vi "Main Controler.vi"() -> ()   [LabVIEW 2022 SP3]
uses:
  Controls/Display Loop ctl.ctl
  Loop.ctl
  Controls/ALL Health.ctl
  cd6b9e46-59f8-41b3-9490-225fb67d1ba0.vi
  1b3de88b-dec3-4abe-965c-7ad6896efe13.vi
  9936e6a7-bc3d-4afe-8410-a89b98546ed9.vi
  d1ab7018-2df1-4ffb-970b-af0fe01cb293.vi
  e0eb6b05-03bb-4813-a05d-282ab3cd3a22.vi
  ecf1675c-338f-4a89-ac69-4cdab471b100.vi
  ca0a8722-a5c4-4655-b82c-d313b5c34e14.vi
  c976ff62-2192-4a2c-b2cc-abbf70db85cd.vi
  943ba9a9-8a3c-4e90-9b72-098ad84989a2.vi
  675b6325-e57b-42b8-b386-55e59851567e.vi
  d7703bda-d248-4b1e-9ee4-ce44b9949d59.vi
  ad1d9b89-0aa4-4254-89c1-c2ee87c320aa.vi
  35d283f9-0e0c-41d3-ba70-7538f373975d.vi
  c92325a5-4571-45f9-94fe-0f0a9663467d.vi
  6D_Global.vi
  8e23ed98-7719-4f36-858a-146910f058b4.vi
panel:
  out "OUT_D_PT":dbl format="%.2g"
  out "AI 1kHZ HS":bool
  out "D_PT_2":dbl format="%.2f"
  out "D_RTD_1":dbl format="%#.2g"
  out "D_PT_1":dbl format="%.2g"
  out "M_RTD_1":dbl format="%#.2g"
  out "M_PT_1":dbl format="%.2g"
  out "OUT_D_RTD":dbl format="%#.2g"
  out "IN_D_RTD":dbl format="%#.2g"
  out "D_RTD_2":dbl format="%#.2g"
  out "IN_D_PT":dbl format="%.2g"
  out "AI 20kHZ HS":bool
  out "Vdc":dbl
  out "Ic_Unbal":bool
  out "Ib_Unbal":bool
  out "Ia_Unbal":bool
  out "Overall Unbal":bool
  out "Ic_G":bool
  out "Ib_G":bool
  out "Ia_G":bool
  out "IDC":bool
  out "Ic":bool
  out "Ib":bool
  out "Ia":bool
  in  "Unbal Threshold":dbl
  in  "10 SAMPLES _G":dbl
  in  "2 SAMPLES_G":dbl
  in  "Log Period":dbl=900.0
  out "DO HS":bool
  out "Idc_G":dbl
  out "Vdc_G":dbl
  out "Hc_G":bool=TRUE
  out "Hb_G":bool=TRUE
  out "Ha_G":bool=TRUE
  out "Ic_G":dbl
  out "Ib_G":dbl
  out "Ia_G":dbl
  out "Vca_G":dbl
  out "Vbc_G":dbl
  out "Vab_G":dbl
  in  "Update RTD Offset_G 2":bool
  in  "V-Ref_B":dbl=3.306
  in  "RTD 6 Offset_B":dbl=1.432
  in  "RTD 5 Offset_B":dbl=1.432
  in  "RTD 4 Offset_B":dbl=1.427
  in  "RTD 3 Offset_B":dbl=1.421
  in  "RTD 2 Offset_B":dbl=1.429
  in  "RTD 1 Offset_B":dbl=1.429
  out "RTD  6":dbl format="%#_f "
  out "RTD  5":dbl format="%#_f "
  out "RTD  4":dbl format="%#_f "
  out "RTD  3":dbl format="%#_f "
  out "RTD  2":dbl format="%#_f "
  out "RTD  1":dbl format="%#_f "
  out "AI HS":bool
  in  "Update RTD Offset_G":bool
  in  "V-Ref_G":dbl=3.306
  in  "RTD 6 Offset_G":dbl=1.432
  in  "RTD 5 Offset_G":dbl=1.432
  in  "RTD 4 Offset_G":dbl=1.427
  in  "RTD 3 Offset_G":dbl=1.421
  in  "RTD 2 Offset_G":dbl=1.429
  in  "RTD 1 Offset_G":dbl=1.429
  out "LOG HS":bool
  in  "Datalog Prefix":string
  in  "Activate Task 2":T1
  in  "Update RTD Offset":bool
  in  "V-Ref":dbl=3.29
  in  "RTD 6 Offset":dbl
  in  "RTD 5 Offset":dbl
  in  "RTD 4 Offset":dbl
  in  "RTD 3 Offset":dbl
  in  "RTD 2 Offset":dbl
  in  "RTD 1 Offset":dbl
  out "DAQ Idc":dbl
  out "M-STATE FB":bool
  out "RUN DUTY RATIO":dbl format="%#_6f"
  out "IDC":dbl format="%#_f "
  out "Idc M-Avg":dbl format="%#_f "
  out "VOLTAGE SPEED":dbl format="%#_f "
  out "HALL SPEED":dbl format="%#_f "
  out "SECTOR":dbl format="%#_f "
  out "VDC":dbl format="%#_f "
  out "DIRECTION":string
  out "RUN ACK":bool
  out "Hc":bool=TRUE
  out "Hb":bool=TRUE
  out "Ha":bool=TRUE
  out "Ic":dbl
  out "Ib":dbl
  out "Ia":dbl
  out "Vca":dbl
  out "Vbc":dbl
  out "Vab":dbl
  out "Power Failure":bool
  out "M-S Failure":bool=TRUE
  out "PPSU Alarm":bool
  out "Over Voltage":bool
  out "Over Current":bool
  out "Over Power":bool
  in  "IDC":dbl
  in  "10 SAMPLES":dbl
  in  "2 SAMPLES":dbl
  out "RUN DUTY RATIO":dbl format="%#_6f"
  out "M-STATE FB":bool
  out "IDC":dbl format="%#_f "
  out "Idc M-Avg":dbl format="%#_f "
  out "VOLTAGE SPEED":dbl format="%#_f "
  out "HALL SPEED":dbl format="%#_f "
  out "SECTOR":dbl format="%#_f "
  out "VDC":dbl format="%#_f "
  out "DIRECTION":string
  out "RUN ACK":bool
  in  "PPSU IP":u8[](array[numeric])=[192, 168, 1, 120]
  in  "Enable PPSU":bool
  out "PPSU HS":bool
  in  "MS initialise":bool
  in  "PPSU ACK Alarm":bool
  out "PPSU 2 HS":bool
  out "VOLTAGE":string
  out "CURRENT":string
  out "POWER":string
  in  "DC OFF 2":bool
  in  "DC ON 2":bool
  in  "Motor Off":bool
  in  "DC OFF":bool
  in  "Motor On":bool
  in  "DC ON":bool
  out "E3-L-RTD":bool
  out "E3-A-RTD":bool
  out "E2-L-RTD":bool
  out "E5 - RTD":bool
  out "E2-RTD":bool
  out "E1-RTD":bool
  out "E1-MFB":bool
  out "E2-MFB":bool
  out "E2-A-MFB":bool
  out "E2-L-MFB":bool
  out "E3-A-MFB":bool
  out "E3-L-MFB":bool
  in  "Disconnect Drive":bool
  in  "Connect Drive":bool
  in  "Port Config File":path=path "C:/Users/Karishmaa- LabVIEW/Desktop/V1.0 Drive6_Control_Monitor/Data/Port ID Config .csv"
  in  "GD ON":bool
  in  "GD OFF":bool
  out "RTD  6":dbl format="%#_f "
  out "RTD  5":dbl format="%#_f "
  out "RTD  4":dbl format="%#_f "
  out "RTD  3":dbl format="%#_f "
  out "RTD  2":dbl format="%#_f "
  out "RTD  1":dbl format="%#_f "
  out "RTD 6":dbl format="%#_f "
  out "RTD  5":dbl format="%#_f "
  out "RTD  4":dbl format="%#_f "
  out "RTD 3":dbl format="%#_f "
  out "RTD  2":dbl format="%#_f "
  out "RTD  1":dbl format="%#_f "
  in  "Update PPSU settings":bool
  in  "PPSU-SETTINGS":T2 {"SET POWER" format="%#_g W"; "SET CURRENT" format="%#_g A"; "SET VOLT" format="%#_g V"; "OPP" format="%#_g W"; "OCP" format="%#_g A"; "OVP" format="%#_g V"}
  in  "Update E1A":bool
  in  "MOTOR":T3 {"M-STATE" format="%#_g "; "DC LIMIT" format="%#_g A"; "RAMP DOWN" format="%#_g Sec"; "RAMP UP" format="%#_g Sec"; "SWITCHING FREQ" format="%#_g Hz"}
  in  "DO CONFIG":cluster{"NAME":string, "CHANNEL NAME":tag}[](array[cluster])
  out "RTD  30":dbl format="%#_f "
  out "RTD  29":dbl format="%#_f "
  out "RTD  28":dbl format="%#_f "
  out "RTD  27":dbl format="%#_f "
  out "RTD  26":dbl format="%#_f "
  out "RTD  25":dbl format="%#_f "
  out "RTD  24":dbl format="%#_f "
  out "RTD  23":dbl format="%#_f "
  out "RTD  22":dbl format="%#_f "
  out "RTD  21":dbl format="%#_f "
  out "RTD  20":dbl format="%#_f "
  out "RTD  19":dbl format="%#_f "
  out "RTD  18":dbl format="%#_f "
  out "RTD  17":dbl format="%#_f "
  out "RTD  16":dbl format="%#_f "
  out "RTD  15":dbl format="%#_f "
  out "RTD  14":dbl format="%#_f "
  out "RTD  13":dbl format="%#_f "
  out "RTD  12":dbl format="%#_f "
  out "RTD  11":dbl format="%#_f "
  out "RTD  10":dbl format="%#_f "
  out "RTD  9":dbl format="%#_f "
  out "RTD  8":dbl format="%#_f "
  out "RTD  7":dbl format="%#_f "
  out "FREQUENCY  2":dbl format="%#_f "
  out "VDC  3":dbl format="%#_f "
  out "IDC  3":dbl format="%#_f "
  out "MOV-IDC  2":dbl format="%#_f "
  out "M-STATE  2":dbl format="%#_f "
  out "DIRECTION  2":string
  out "SPEED 5":dbl format="%#_f r/m"
  out "RUN ACK 5":bool
  out "FREQUENCY  2":dbl format="%#_f "
  out "VDC 2":dbl format="%#_f "
  out "IDC  3":dbl format="%#_f "
  out "MOV-IDC  2":dbl format="%#_f "
  out "M-STATE  2":dbl format="%#_f "
  out "DIRECTION  2":string
  out "SPEED 4":dbl format="%#_f r/m"
  out "RUN ACK 4":bool
  out "FREQUENCY  2":dbl format="%#_f "
  out "VDC  2":dbl format="%#_f "
  out "IDC 2":dbl format="%#_f "
  out "MOV-IDC  2":dbl format="%#_f "
  out "M-STATE  2":dbl format="%#_f "
  out "DIRECTION  2":string
  out "SPEED 3":dbl format="%#_f r/m"
  out "RUN ACK 3":bool
  out "FREQUENCY  2":dbl format="%#_f "
  out "VDC  2":dbl format="%#_f "
  out "IDC  2":dbl format="%#_f "
  out "MOV-IDC  2":dbl format="%#_f "
  out "M-STATE  2":dbl format="%#_f "
  out "DIRECTION  2":string
  out "SPEED 2":dbl format="%#_f r/m"
  out "RUN ACK 2":bool
  in  "Start DAQ":bool
  in  "Stop DAQ":bool
  in  "Start Log":bool
  in  "Stop Log":bool
  in  "Continuous Log?":bool
  in  "Activate Task":T4
  in  "Exit":bool
  # "DRIVE PARMETERS SETTINGS"
  # "*Select section to set parameters"
  # "DRIVE-3- CONTROL & MONITORING SCREEN"
  # "VERSION 1.0"
  # "ACTIVE PORTS"
  # "MOTOR FEEDBACK DATA"
  # "PPSU DATA"
  # "PPSU HS"
  # "DAQ & LOG SETTINGS"
  # "MOTOR"
  # "GENERATOR"
  # "PROPULSION"
  # "PPSU-2 HS"
  # "PROTECTION"
  # "MCU RESET"
  # "E2-ATF MOTOR FEEDBACK DATA"
  # "E2-LOX MOTOR FEEDBACK DATA"
  # "E3-ATF MOTOR FEEDBACK DATA"
  # "E3-ATF MOTOR FEEDBACK DATA"
  # "E2-ATF TEMPRATURE DATA"
  # "E2-LOX TEMPRATURE DATA"
  # "E3-ATF TEMPRATURE DATA"
  # "E3-LOX TEMPRATURE DATA"
  # "BEARING TEMPRATURE DATA"
  # "E1-LOX"
  # "E1-ATF"
  # "E2-ATF"
  # "E2-LOX"
  # "E3-ATF"
  # "E3-LOX"
  # "GENERATOR FEEDBACK DATA"
  # "GENERATOR TEMPRATURE DATA"
  # "MOTOR TEMPRATURE DATA"
  # "GNIKUL"
  # "Drive 1"
  # "Drive 2"
  # "Drive 3"
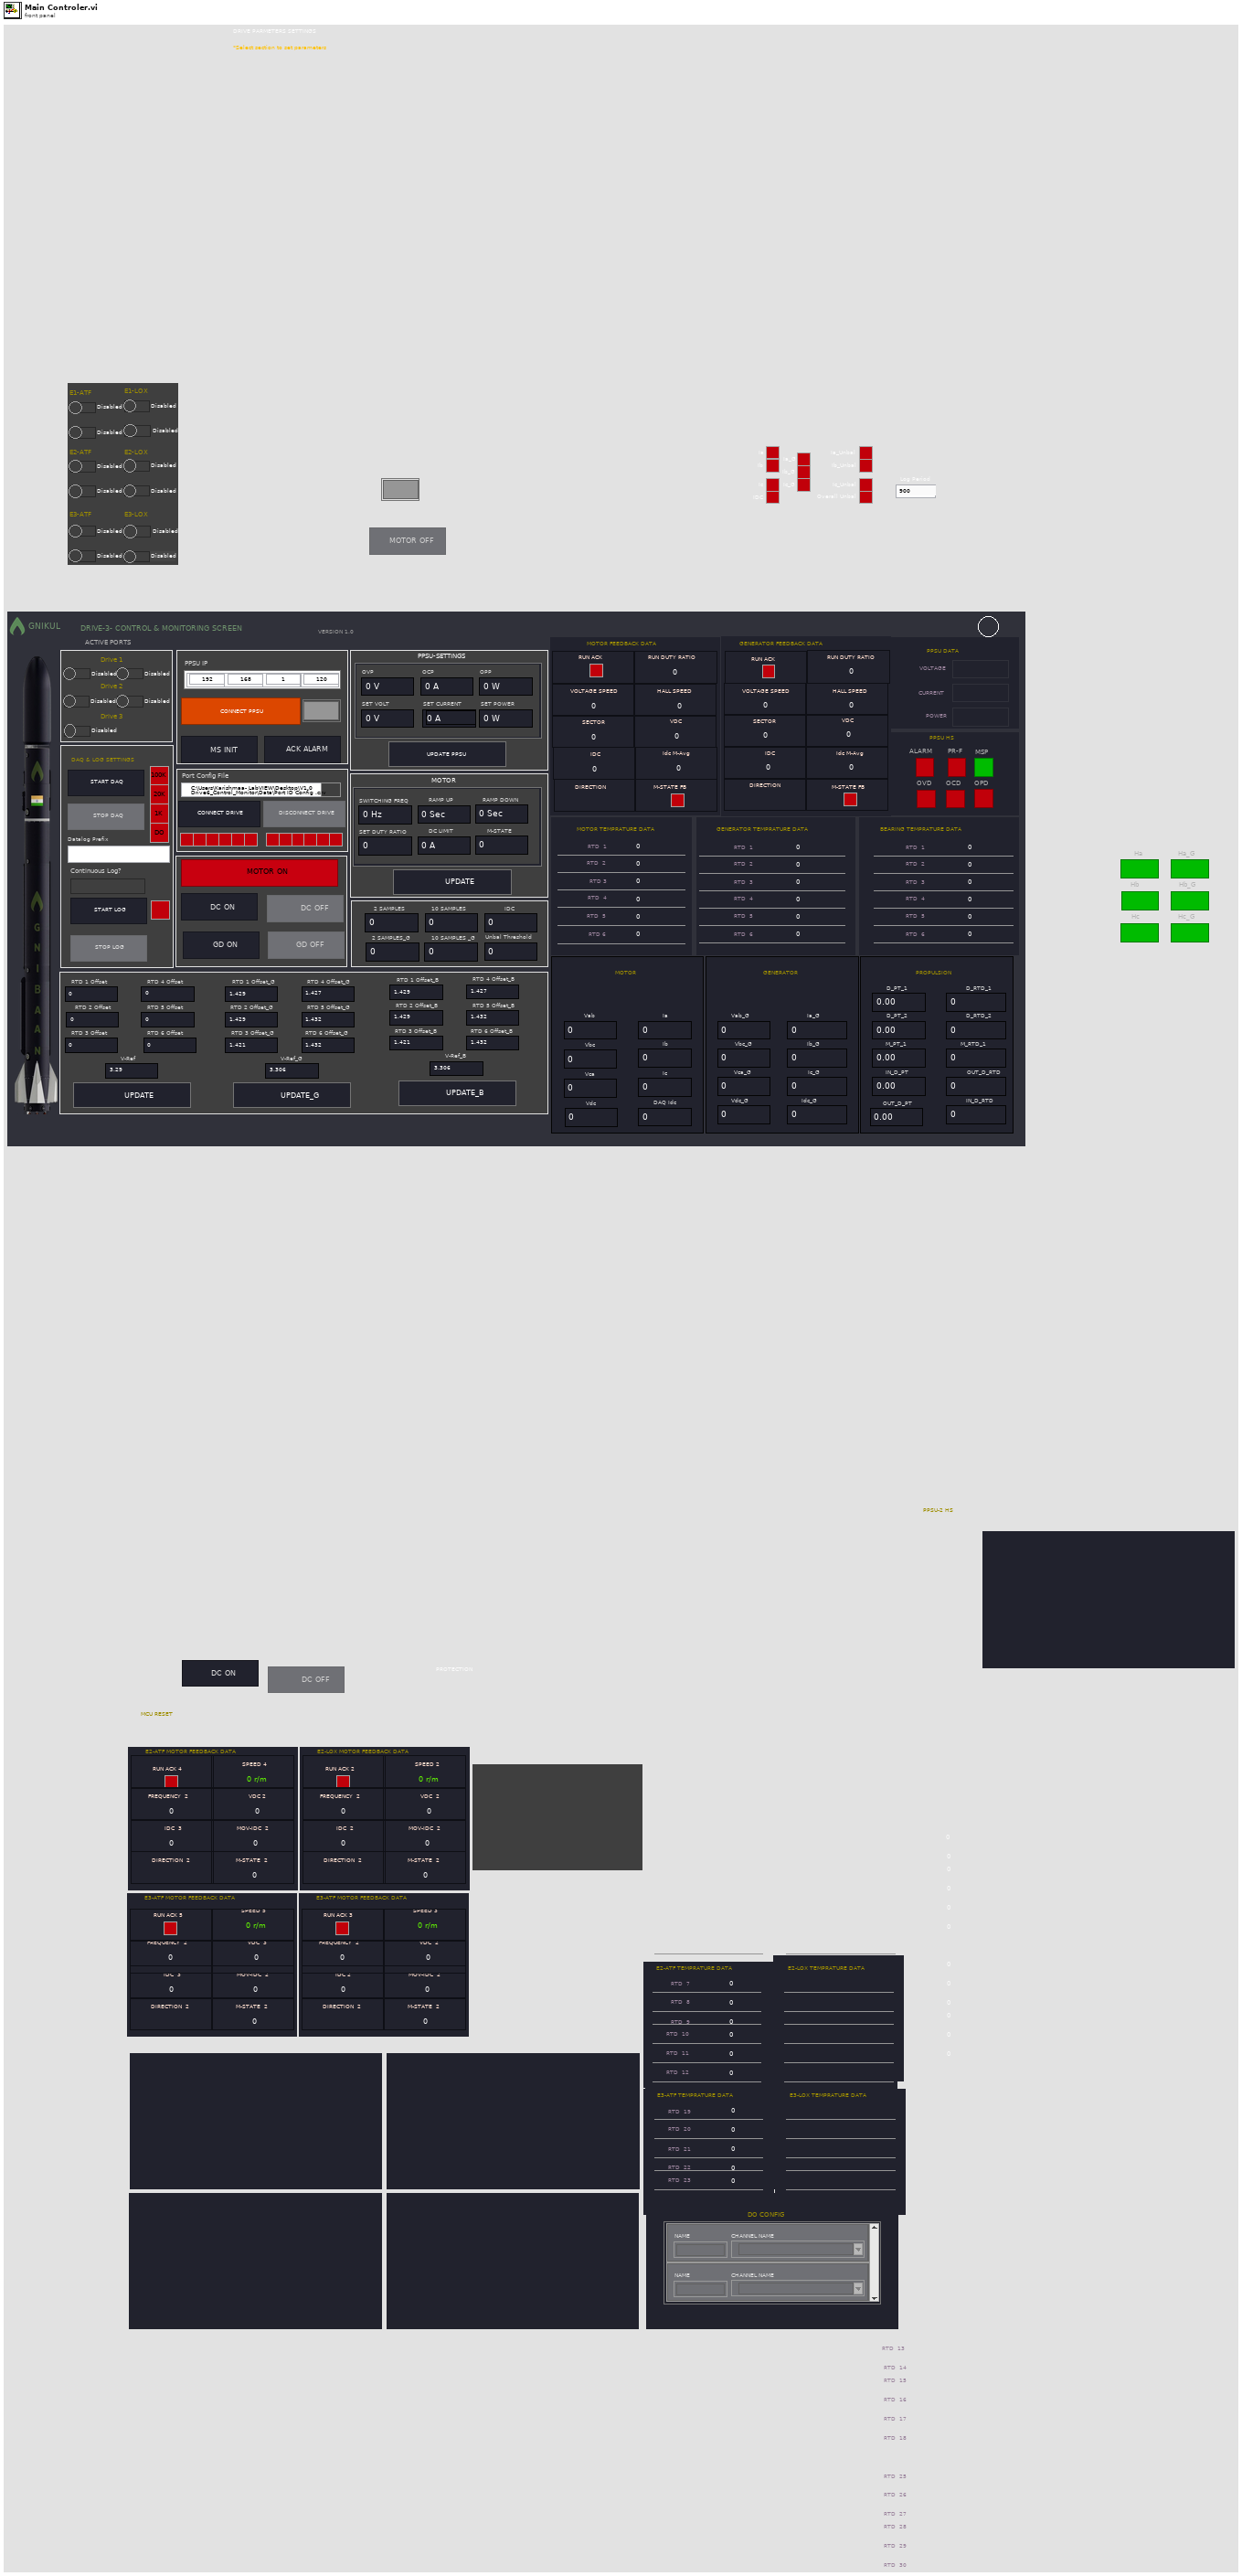
[diagram p1: front panel]
types:
  T1 = cluster{"ETH_1":bool, "ETH_2":bool, "ETH_3":bool, "ETH_4":bool, "ETH_5":bool, "ETH_6":bool, "ETH_7":bool, "ETH_8":bool, "ETH_9":bool, "ETH_10":bool, "ETH_11":bool, "ETH_12":bool}
  T2 = cluster{"OPP":dbl, "OVP ":dbl, "OCP":dbl, "SET VOLT":dbl, "SET CURRENT":dbl, "SET POWER":dbl}
  T3 = cluster{"SWITCHING FREQ":dbl, "RAMP UP":dbl, "RAMP DOWN":dbl, "SET DUTY RATIO":dbl, "DC LIMIT":dbl, "M-STATE":dbl}
  T4 = cluster{"ETH_1":bool, "ETH_2":bool, "ETH_3":bool, "ETH_4":bool, "ETH_3 2":bool}
  T5 = enum16{"Init", "Read 'All'", "Read 'n'", "Read '1'", "Write '1'", "Write 'n'", "Write 'All'"}
  T6 = typedef "Display Loop ctl.ctl" = enum16{"Motor", "RTD", "All Health", "PPSU"}
  T7 = enum16{"Init", "EnQ '1'", "EnQ 'n'", "EnQ Opp", "DeQ", "Flush", "Close"}
  T8 = cluster{"Device information":string[], "Device information array":string[][], "PPSU IP String":string}
  T9 = cluster{"ETH_1":bool, "ETH_2":bool, "ETH_3":bool, "ETH_4":bool, "ETH_5":bool}
  T10 = enum8{"Enabled", "Disabled", "Disabled and Grayed Out"}[]
  T11 = typedef "All Queue Ref.ctl" = cluster{"MFB":cluster{"ETH_1 E1A_MFB":refnum<queue>, "ETH_3 E1L_MFB":refnum<queue>, "ETH_5 E2A_MFB":refnum<queue>, "ETH_7 E2L_MFB":refnum<queue>, "ETH_9 E3A_MFB":refnum<queue>, "ETH_11 E3L_MFB":refnum<queue>}, "RTD":cluster{"ETH_2 E1A_RTD ":refnum<queue>, "ETH_4 E1L_RTD ":refnum<queue>, "ETH_6 E2A_RTD ":refnum<queue>, "ETH_8 E2L_RTD ":refnum<queue>, "ETH_10 E3A_RTD ":refnum<queue>, "ETH_12 E3L_RTD ":refnum<queue>}, "DO DAQ":refnum<queue>, "PPSU 1 Data":refnum<queue>, "PPSU 2 Data":refnum<queue>, "AI DAQ RMS DATA":refnum<queue>, "AI DAQ RAW DATA":refnum<queue>, "DI DAQ":refnum<queue>, "AI Propulsion RAW DAQ Data":refnum<queue>, "AI Propulsion RMS DAQ Data":refnum<queue>, "AI Vibration DAQ Data":refnum<queue>}
  T12 = typedef "ALL Health.ctl" = enum16{"AI HS", "AI Vibration HS", "AI Propulsion HS", "DO HS", "Datalog HS", "PPSU HS", "ETH_1 DAQ", "ETH_1 RTD", "ETH_2 DAQ", "ETH_2 RTD", "ETH_5 RTD"}
  T13 = cluster{"Run ACK":bool, "RDR":dbl, "Sector":dbl, "Halls Speed":dbl, "Mode":bool, "Voltage Speed":dbl, "Direction":string, "IDC":dbl, "Movable average":dbl, "VDC":dbl}
  T14 = cluster{"Alarm":bool, "Power Fail":bool, "OVD":bool, "OCD":bool, "OPD":bool, "MSP":bool}
  T15 = typedef "Loop.ctl" = enum16{"ETH_1", "ETH_2", "ETH_3", "ETH_4", "ETH_5", "ETH_6", "ETH_7", "ETH_8", "ETH_9", "ETH_10", "ETH_11", "ETH_12"}
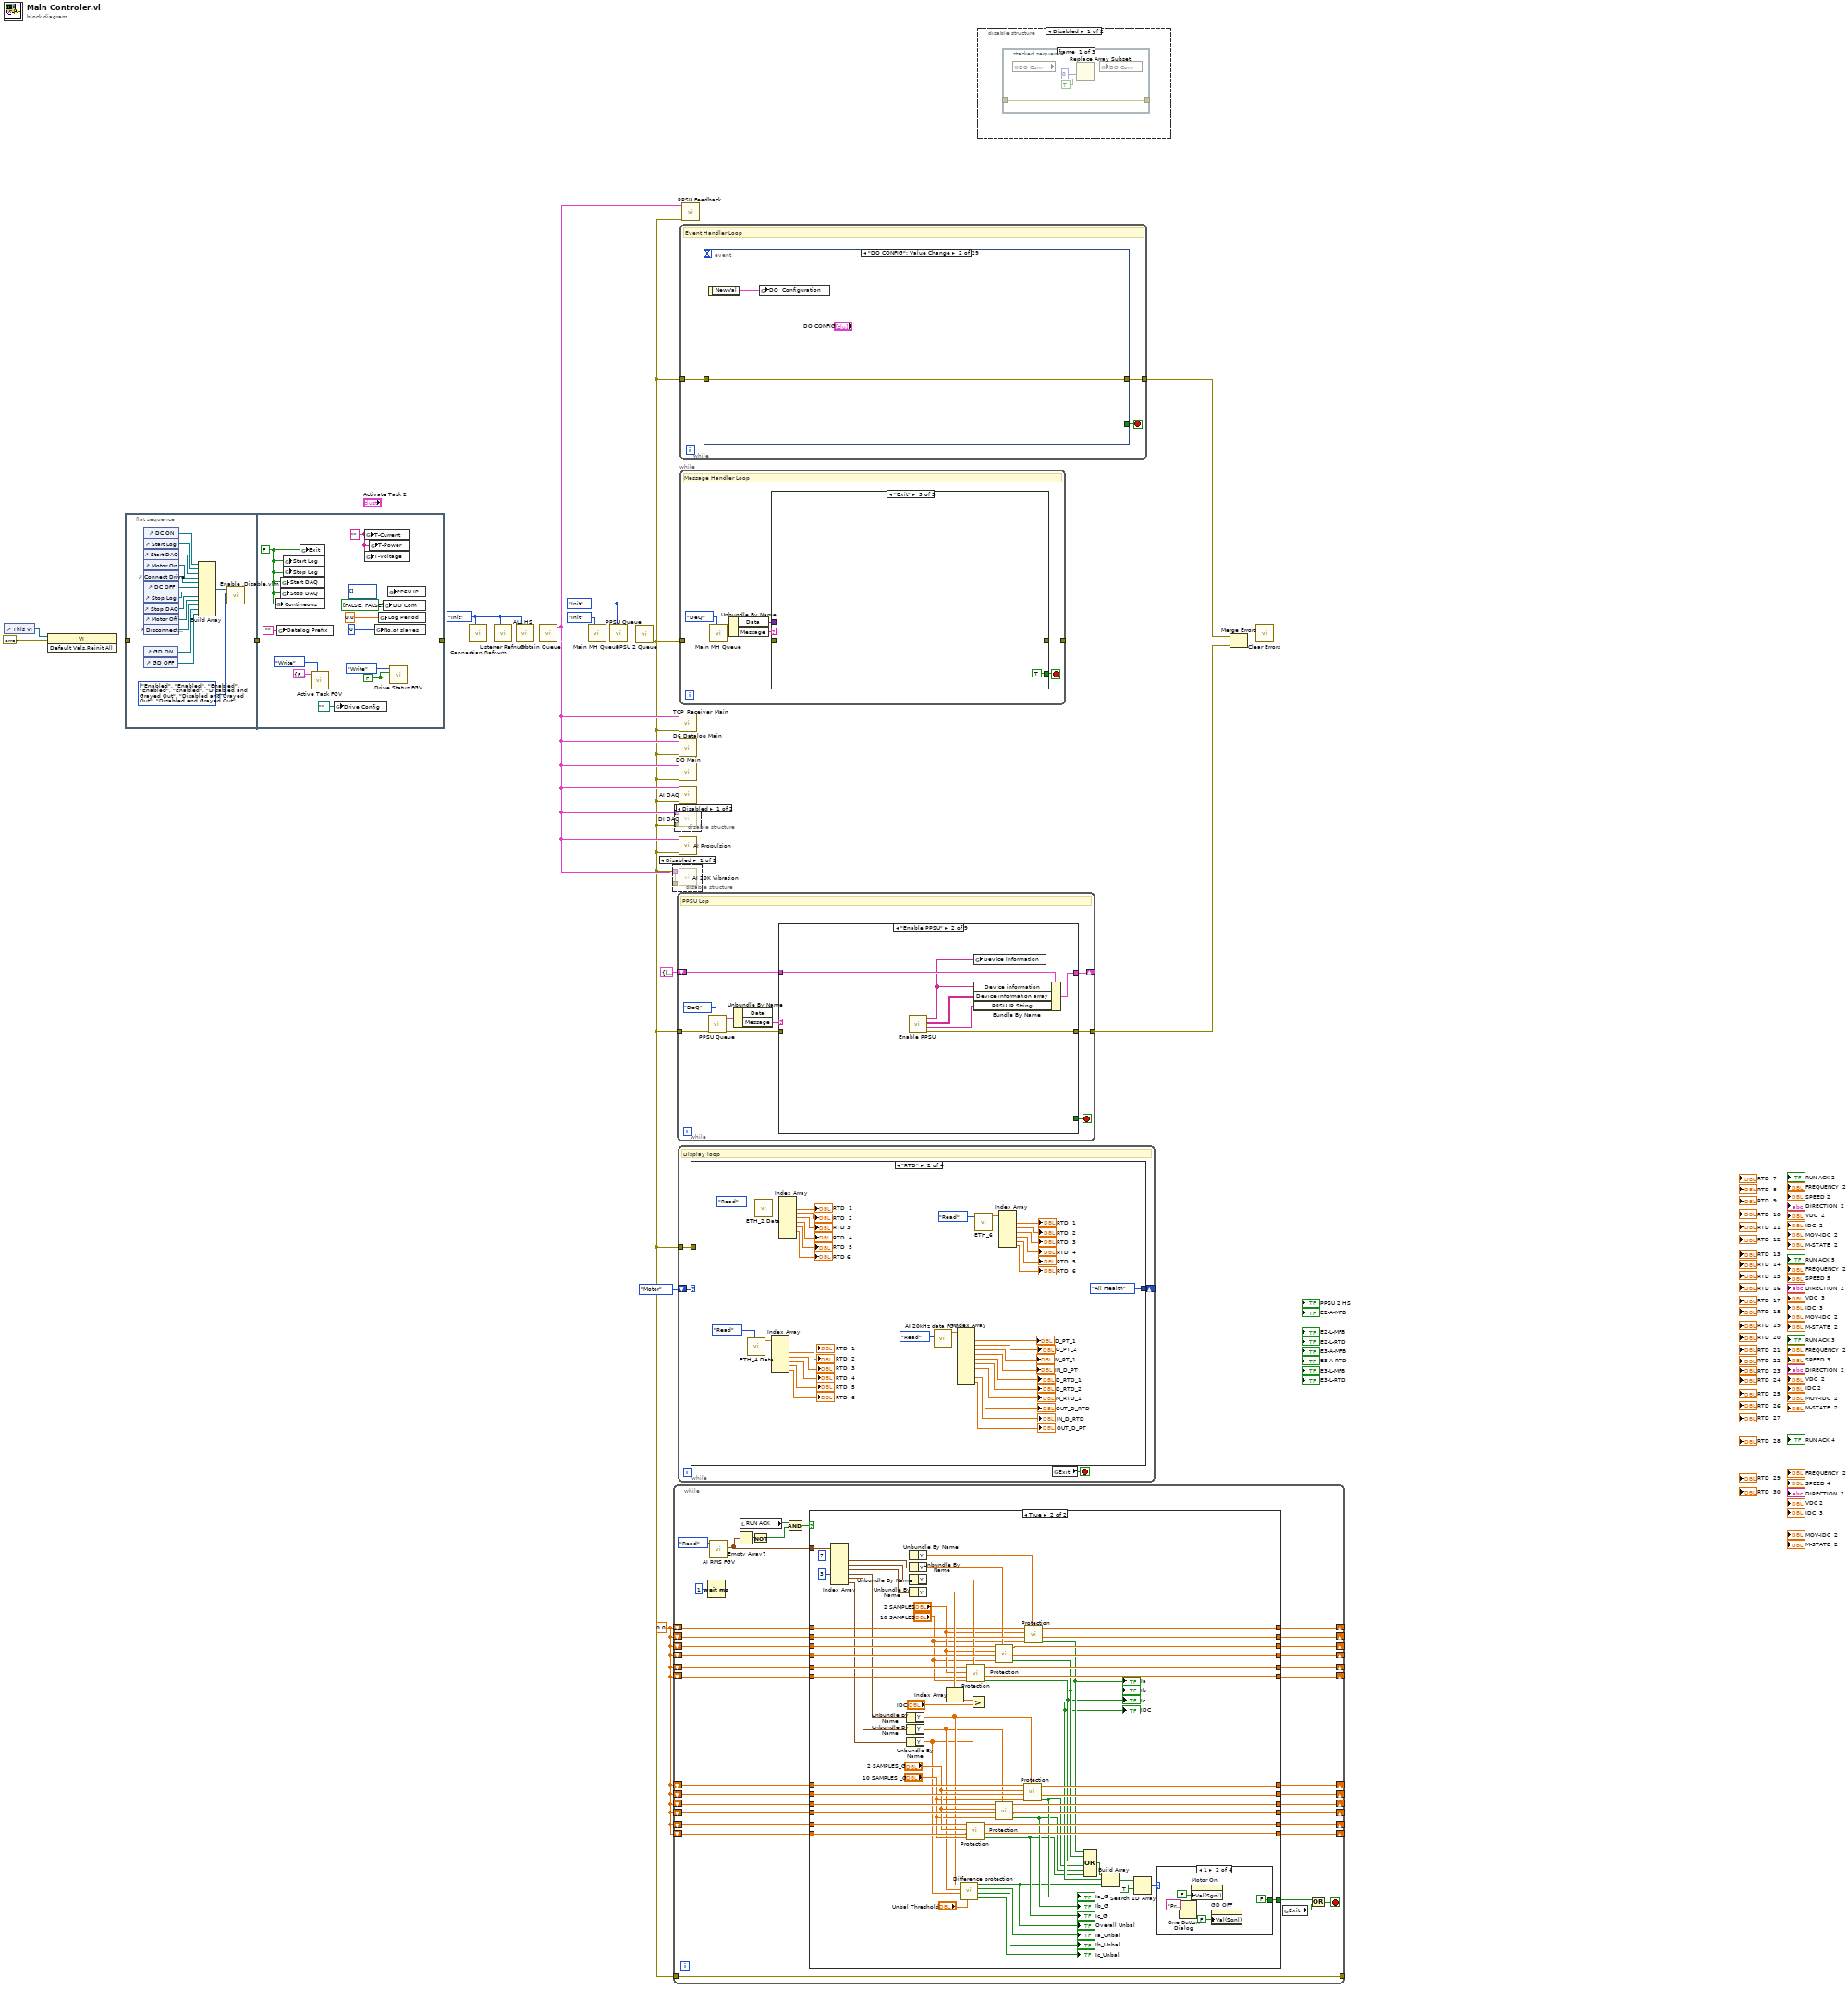
[diagram p0: block diagram]
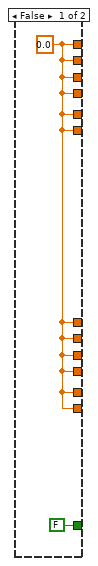
[diagram p4: hidden frame]
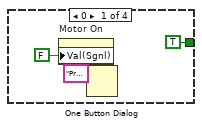
[diagram p5: hidden frame]
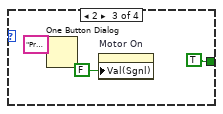
[diagram p6: hidden frame]
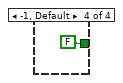
[diagram p7: hidden frame]
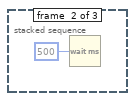
[diagram p8: hidden frame]
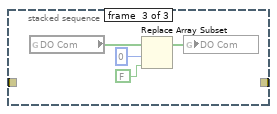
[diagram p9: hidden frame]
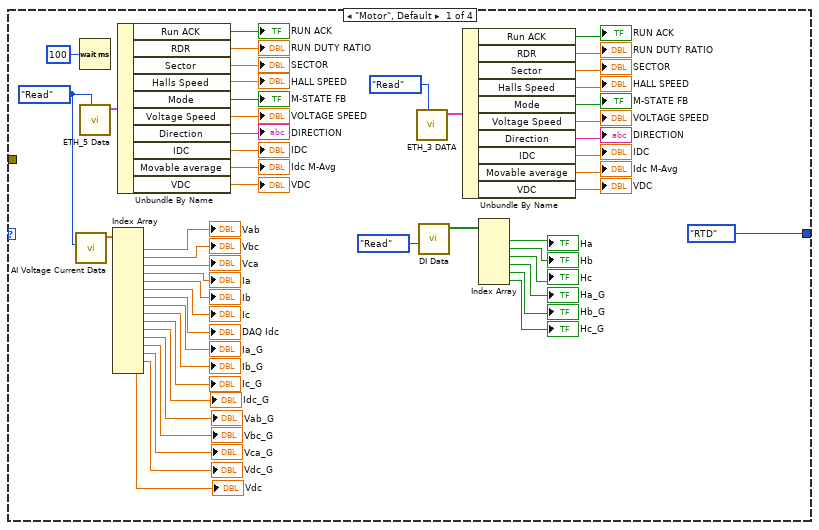
[diagram p11: hidden frame]
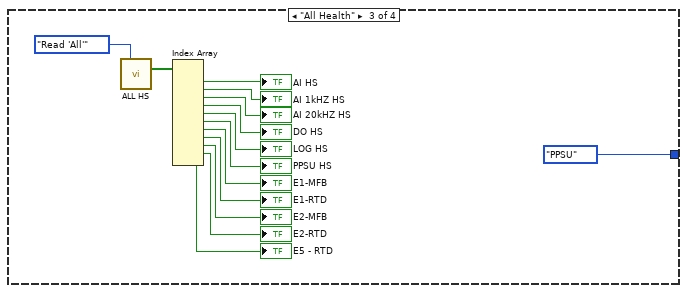
[diagram p12: hidden frame]
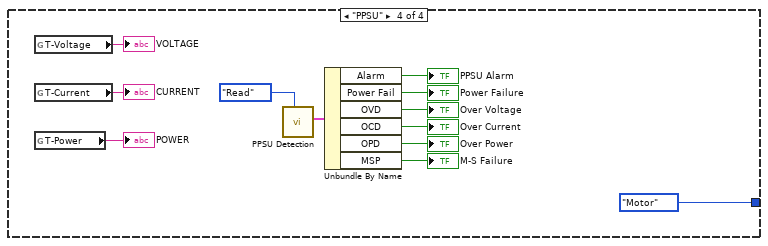
[diagram p13: hidden frame]
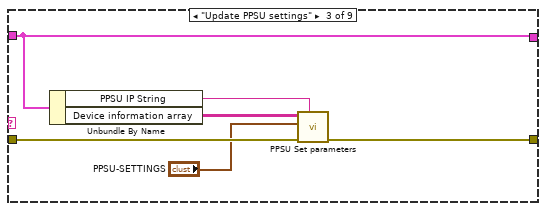
[diagram p15: hidden frame]
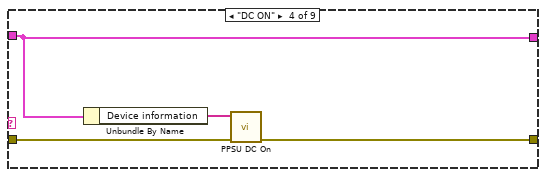
[diagram p16: hidden frame]
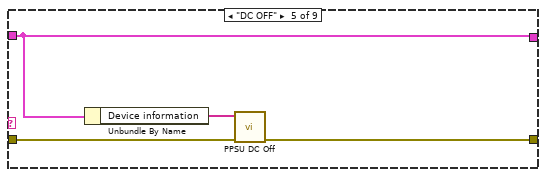
[diagram p17: hidden frame]
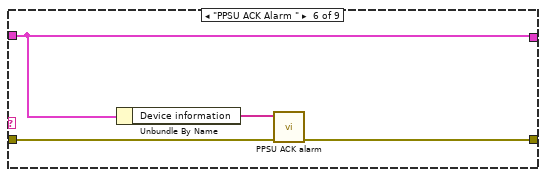
[diagram p18: hidden frame]
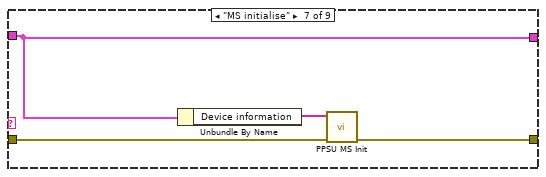
[diagram p19: hidden frame]
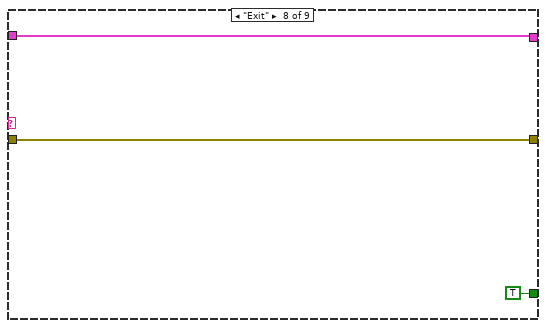
[diagram p20: hidden frame]
diagram:
  w3 = 0.0 ("Trigger 2 out")
  w4 = T5."Init" ("Option")
  w5 = T7."Init" ("Option")
  n1 = control-ref of="This VI"() -> (w22:refnum<vi>)
  n2 = invoke on="Invoke Node" class="VI" method="Default Vals.Reinit All"(reference=w22, error in=errorcluster {"status"=FALSE, "code"=0, "source"=""}) -> (error out=w21:errorcluster)  [unwired: 1 in, 2 out]
  n3 = flat-sequence {
    tunnel: w21 -> [w24]
    tunnel: [w24] -> w11
    tunnel: [w51] -> w10
    tunnel: w11 -> [w51]
    frame #0 {
      w27 = T10 [enum."Enabled", enum."Enabled", enum."Enabled", enum."Enabled", enum."Enabled", enum."Disabled and Grayed Out", enum."Disabled and Grayed Out", enum."Disabled and Grayed Out", enum."Disabled and Grayed Out", enum."Disabled and Grayed Out", enum."Enabled", enum."Disabled and Grayed Out"] items=["Enabled", "Disabled", "Disabled and Grayed Out"] ("Disabled")
      n4 = control-ref of="GD ON"() -> (w26:refnum<vi>)
      n5 = control-ref of="GD OFF"() -> (w25:refnum<vi>)
      n6 = control-ref of="DC ON"() -> (w38:refnum<vi>)
      n7 = control-ref of="Start Log"() -> (w37:refnum<vi>)
      n8 = control-ref of="Start DAQ"() -> (w36:refnum<vi>)
      n9 = control-ref of="Motor On"() -> (w35:refnum<vi>)
      n10 = control-ref of="Connect Drive"() -> (w34:refnum<vi>)
      n11 = control-ref of="DC OFF"() -> (w29:refnum<vi>)
      n12 = control-ref of="Stop Log"() -> (w30:refnum<vi>)
      n13 = control-ref of="Stop DAQ"() -> (w31:refnum<vi>)
      n14 = control-ref of="Motor Off"() -> (w32:refnum<vi>)
      n15 = control-ref of="Disconnect Drive"() -> (w33:refnum<vi>)
      n16 = Build Array(w38, w37, w36, w35, w34, w29, w30, w31, w32, w33, w26, w25) -> (w28:refnum<vi>[])
      n17 = call "Enable ,Disable.vim"("Data"=w27, "Ref"=w28) -> ()  [unwired: 10 in]
    }
    frame #1 {
      w41 = FALSE ("Connect Drive")
      w49 = "" ("T-Current")
      w39 = FALSE ("Exit")
      n18 = global write "6D_Global.vi" "Contineous"(w39) -> ()
      n19 = global write "6D_Global.vi" "Datalog Prefix"("" ("Datalog Prefix")) -> ()
      n20 = global write "6D_Global.vi" "Start DAQ"(w39) -> ()
      n21 = global write "6D_Global.vi" "Stop DAQ"(w39) -> ()
      n22 = global write "6D_Global.vi" "Start Log"(w39) -> ()
      n23 = global write "6D_Global.vi" "Stop Log"(w39) -> ()
      n24 = global write "6D_Global.vi" "Exit"(w39) -> ()
      n25 = call "Active Task FGV.vi"("Write/Read"=enum16{"Write", "Read"}."Write", "Activate Task"=T9 {"ETH_1"=FALSE, "ETH_2"=FALSE, "ETH_3"=FALSE, "ETH_4"=FALSE, "ETH_5"=FALSE}) -> ()  [unwired: 8 in, 2 out]
      n26 = global write "6D_Global.vi" "Drive Config"(path "" ("Drive Config")) -> ()
      n27 = global write "6D_Global.vi" "T-Current"(w49) -> ()
      n28 = global write "6D_Global.vi" "T-Voltage"(w49) -> ()
      n29 = global write "6D_Global.vi" "T-Power"(w49) -> ()
      n30 = global write "6D_Global.vi" "No.of slaves"(u8 0 ("No.of slaves")) -> ()
      n31 = global write "6D_Global.vi" "Log Period"(0.0 ("Log Period")) -> ()
      n32 = global write "6D_Global.vi" "DO Com"(bool[] [FALSE, FALSE] ("DO Com")) -> ()
      n33 = global write "6D_Global.vi" "PPSU IP"(u8[] [] ("PPSU IP")) -> ()
      n34 = call "Drive Status FGV.vi"("Disconnect Drive"=w41, "Connect Drive"=w41, "Enum"=enum16{"Read", "Write"}."Write") -> ()  [unwired: 6 in, 3 out]
    }
  }
  n35 = call "Connection Refnum.vi"("Option"=w4, "error in"=w10) -> ("error out"=w9:errorcluster)  [unwired: 11 in, 2 out]
  n36 = call "Listener Refnum.vi"("Option"=w4, "error in"=w9) -> ("error out"=w8:errorcluster)  [unwired: 11 in, 2 out]
  n37 = call "ALL HS.vi"("Option"=w4, "error in"=w8) -> ("error out"=w7:errorcluster)  [unwired: 11 in, 2 out]
  n38 = call "Obtain Queue.vi"("error out"=w7) -> ("errorout"=w18:errorcluster, "All Queue"=w2:T11)  [unwired: 9 in]
  n39 = call "Main MH Queue.vi"("Option"=T7."Init", "error in (no error)"=w18) -> ("error out"=w15:errorcluster)  [unwired: 8 in, 1 out]
  n40 = call "PPSU Queue.vi"("Option"=w5, "error in"=w15) -> ("error out"=w6:errorcluster)  [unwired: 8 in, 1 out]
  n41 = call "PPSU 2 Queue.vi"("Option"=w5, "error in"=w6) -> ("error out"=w1:errorcluster)  [unwired: 8 in, 1 out]
  n42 = disable-structure shown="Disabled" {
    disable-tunnel: w2 -> [w53 _]
    disable-tunnel: w1 -> [w52 _]
    frame Disabled {
      n43 = call "AI 20K Vibration.vi"("error in (no error)"=w52, "All Queue"=w53) -> ()  [unwired: 9 in, 1 out]
    }
    frame Enabled {
    }
  }
  n44 = while {
    shift-right: [w87] -> _
    shift-left: w3 -> [w81]
    shift-right: [w86] -> _
    shift-left: w3 -> [w80]
    shift-right: [w85] -> _
    shift-left: w3 -> [w79]
    shift-right: [w84] -> _
    shift-left: w3 -> [w78]
    shift-right: [w83] -> _
    shift-left: w3 -> [w77]
    shift-right: [w82] -> _
    shift-left: w3 -> [w76]
    tunnel: w1 -> [w73]
    tunnel: [w73] -> _
    shift-right: [w55] -> _
    shift-left: w3 -> [w61]
    shift-right: [w56] -> _
    shift-left: w3 -> [w62]
    shift-right: [w57] -> _
    shift-left: w3 -> [w63]
    shift-right: [w58] -> _
    shift-left: w3 -> [w64]
    shift-right: [w59] -> _
    shift-left: w3 -> [w65]
    shift-right: [w60] -> _
    shift-left: w3 -> [w66]
    stop <- w70 stop-if-true
    n45 = Wait (ms)(milliseconds to wait=u32 1) -> ()  [unwired: 1 out]
    n46 = call "AI RMS FGV.vi"("Enum"=enum16{"Read", "Write"}."Read") -> ("RMS value waveforms"=w74:waveform(dbl)[])  [unwired: 9 in, 1 out]
    n47 = Empty Array?(array=w74) -> (empty?=w88:bool)
    n48 = local read "RUN ACK"() -> (w54:bool)
    n49 = Not(x=w88) -> (.not. x?=w67:bool)
    n50 = Compound Arithmetic op=AND(w54, w67) -> (w68:bool)
    n51 = case shown="True" w68 {
      tunnel: w74 -> [_ w154]
      tunnel: [w89 w139] -> w87
      tunnel: [w89 w138] -> w86
      tunnel: [w89 w136] -> w85
      tunnel: [w89 w135] -> w84
      tunnel: [w89 w129] -> w83
      tunnel: [w89 w128] -> w82
      tunnel: w81 -> [_ w141]
      tunnel: w80 -> [_ w140]
      tunnel: w79 -> [_ w134]
      tunnel: w78 -> [_ w133]
      tunnel: w77 -> [_ w131]
      tunnel: w76 -> [_ w130]
      tunnel: [FALSE w124] -> w69
      tunnel: [w89 w113] -> w55
      tunnel: [w89 w114] -> w56
      tunnel: [w89 w115] -> w57
      tunnel: [w89 w116] -> w58
      tunnel: [w89 w121] -> w59
      tunnel: [w89 w122] -> w60
      tunnel: w61 -> [_ w111]
      tunnel: w62 -> [_ w112]
      tunnel: w63 -> [_ w117]
      tunnel: w64 -> [_ w118]
      tunnel: w65 -> [_ w119]
      tunnel: w66 -> [_ w120]
      frame False {
        w89 = 0.0 ("Trigger 2 out")
      }
      frame True {
        n52 = Index Array(array=w154, index #1=7 ("index"), index #5=3 ("index")) -> (element #1=w152:waveform(dbl), element #2=w151:waveform(dbl), element #3=w150:waveform(dbl), element #4=w149:waveform(dbl), element #5=w109:waveform(dbl), element #6=w108:waveform(dbl), element #7=w107:waveform(dbl))  [unwired: 5 in]
        n53 = Unbundle By Name(w109) -> ("Y"=w105:dbl[])
        n54 = Unbundle By Name(w108) -> ("Y"=w104:dbl[])
        n55 = Unbundle By Name(w107) -> ("Y"=w103:dbl[])
        n56 = Unbundle By Name(w152) -> ("Y"=w142:dbl[])
        n57 = Unbundle By Name(w151) -> ("Y"=w137:dbl[])
        n58 = Unbundle By Name(w150) -> ("Y"=w132:dbl[])
        n59 = Unbundle By Name(w149) -> ("Y"=w148:dbl[])
        n60 = Index Array(array=w148) -> (element=w147:dbl)  [unwired: 1 in]
        n61 = call "Difference protection.vi"("Common Threshold"="Unbal Threshold", "RMS Ic"=w103, "RMS Ib"=w104, "RMS Ia"=w105) -> ("Ic Un"=→"Ic_Unbal":bool, "Ib Un"=→"Ib_Unbal":bool, "Ia Un"=→"Ia_Unbal":bool, "Overall"=w94:bool)  [unwired: 4 in]
        "Overall Unbal" <- w94
        n62 = call "Protection.vi"("RMS Value"=w103, "10 Amps"="10 SAMPLES _G", "Trigger 10 times"=w120, "5 Amps"="2 SAMPLES_G", "Trigger 2 times"=w119) -> ("Trigger"=w95:bool, "Trigger 10 out"=w122:dbl, "Trigger 2 out"=w121:dbl)  [unwired: 4 in]
        "Ic_G" <- w95
        n63 = call "Protection.vi"("RMS Value"=w132, "10 Amps"="10 SAMPLES", "Trigger 10 times"=w130, "5 Amps"="2 SAMPLES", "Trigger 2 times"=w131) -> ("Trigger"=w99:bool, "Trigger 10 out"=w128:dbl, "Trigger 2 out"=w129:dbl)  [unwired: 4 in]
        "Ic" <- w99
        n64 = Greater?(x=w147, y="IDC") -> (0:w98:bool)
        "IDC" <- w98
        n65 = call "Protection.vi"("RMS Value"=w104, "10 Amps"="10 SAMPLES _G", "Trigger 10 times"=w118, "5 Amps"="2 SAMPLES_G", "Trigger 2 times"=w117) -> ("Trigger"=w96:bool, "Trigger 10 out"=w116:dbl, "Trigger 2 out"=w115:dbl)  [unwired: 4 in]
        "Ib_G" <- w96
        n66 = call "Protection.vi"("RMS Value"=w137, "10 Amps"="10 SAMPLES", "Trigger 10 times"=w133, "5 Amps"="2 SAMPLES", "Trigger 2 times"=w134) -> ("Trigger"=w100:bool, "Trigger 10 out"=w135:dbl, "Trigger 2 out"=w136:dbl)  [unwired: 4 in]
        "Ib" <- w100
        n67 = call "Protection.vi"("RMS Value"=w105, "10 Amps"="10 SAMPLES _G", "Trigger 10 times"=w112, "5 Amps"="2 SAMPLES_G", "Trigger 2 times"=w111) -> ("Trigger"=w97:bool, "Trigger 10 out"=w114:dbl, "Trigger 2 out"=w113:dbl)  [unwired: 4 in]
        "Ia_G" <- w97
        n68 = call "Protection.vi"("RMS Value"=w142, "10 Amps"="10 SAMPLES", "Trigger 10 times"=w140, "5 Amps"="2 SAMPLES", "Trigger 2 times"=w141) -> ("Trigger"=w101:bool, "Trigger 10 out"=w138:dbl, "Trigger 2 out"=w139:dbl)  [unwired: 4 in]
        "Ia" <- w101
        n69 = Compound Arithmetic op=OR(w101, w100, w99, w97, w96, w95) -> (w146:bool)
        n70 = Build Array(w146, w98, w94) -> (w145:bool[])
        n71 = Search 1D Array(1D array=w145, element=TRUE) -> (index of element=w143:i32)  [unwired: 1 in]
        n72 = case shown="1" w143 {
          tunnel: [TRUE FALSE TRUE FALSE] -> w124
          frame 0 {
            n73 = property on="Motor On" class="Bool (strict)"("Val(Sgnl)"=FALSE ("Value (Signaling)")) -> ()  [unwired: 2 in, 2 out]
            n74 = One Button Dialog(message="Protection Triggered") -> ()  [unwired: 1 in, 1 out]
          }
          frame 1 {
            n75 = One Button Dialog(message="Protection Triggered") -> ()  [unwired: 1 in, 1 out]
            n76 = property on="Motor On" class="Bool (strict)"("Val(Sgnl)"=FALSE ("Value (Signaling)")) -> ()  [unwired: 2 in, 2 out]
            n77 = property on="GD OFF" class="Bool (strict)"("Val(Sgnl)"=FALSE ("Value (Signaling)")) -> ()  [unwired: 2 in, 2 out]
          }
          frame 2 {
            n78 = One Button Dialog(message="Protection Triggered") -> ()  [unwired: 1 in, 1 out]
            n79 = property on="Motor On" class="Bool (strict)"("Val(Sgnl)"=FALSE ("Value (Signaling)")) -> ()  [unwired: 2 in, 2 out]
          }
          frame -1, Default {
          }
        }
      }
    }
    n80 = global read "6D_Global.vi" "Exit"() -> (w71:bool)
    n81 = Or(x=w69, y=w71) -> (x .or. y?=w70:bool)
  }
  n82 = disable-structure shown="Disabled" {
    disable-tunnel: w2 -> [w167 _]
    disable-tunnel: w1 -> [w166 _]
    frame Disabled {
      n83 = call "DI DAQ.vi"("error in"=w166, "All Queue"=w167) -> ()  [unwired: 9 in, 1 out]
    }
    frame Enabled {
    }
  }
  n84 = while {
    tunnel: w1 -> [w173]
    tunnel: [w172] -> w17
    shift-right: [w169] -> _
    shift-left: T8 {"Device information"=[], "Device information array"=[], "PPSU IP String"=""} -> [w170]
    stop <- w168 stop-if-true
    # "PPSU Lop"
    n85 = call "PPSU Queue.vi"("Option"=T7."DeQ", "error in"=w173) -> ("error out"=w171:errorcluster, "Message Out"=w175:cluster{"Message":string, "Data":variant})  [unwired: 8 in]
    n86 = Unbundle By Name(w175) -> ("Message"=w174:string)  [unwired: 1 out]
    n87 = case shown="\"Enable PPSU\"" w174 {
      tunnel: [w177 w184 w189 w192 w196 w201 w205 w208 w212] -> w172
      tunnel: w171 -> [w177 _ w190 w193 w197 w202 w206 w208 w211]
      tunnel: w170 -> [w178 w183 w188 w191 w195 w199 w203 w209 w214]
      tunnel: [w178 w182 w188 w191 w195 w199 w203 w209 w214] -> w169
      tunnel: [_ _ _ _ _ _ _ TRUE _] -> w168
      frame "", Default {
      }
      frame "Enable PPSU" {
        n88 = call "Enable PPSU.vi"() -> ("error Out"=w184:errorcluster, "PPSU IP String"=w180:string, "Device information array"=w181:string[][], "Device information"=w179:string[])  [unwired: 8 in]
        n89 = global write "6D_Global.vi" "Device information"(w179) -> ()
        n90 = Bundle By Name(cluster=w183, "Device information"=w179, "Device information array"=w181, "PPSU IP String"=w180) -> (w182:T8)
      }
      frame "Update PPSU settings" {
        n91 = Unbundle By Name(w188) -> ("PPSU IP String"=w186:string, "Device information array"=w185:string[][])
        n92 = call "PPSU Set parameters.vi"("PPSU IP String"=w186, "Error in"=w190, "Data"="PPSU-SETTINGS", "Device information array"=w185) -> ("Fehler (Ausgang)"=w189:errorcluster)  [unwired: 6 in, 1 out]
      }
      frame "DC ON" {
        n93 = Unbundle By Name(w191) -> ("Device information"=w194:string[])
        n94 = call "PPSU DC On.vi"("Error in"=w193, "Device information"=w194) -> ("Error out"=w192:errorcluster)  [unwired: 8 in, 1 out]
      }
      frame "DC OFF" {
        n95 = Unbundle By Name(w195) -> ("Device information"=w198:string[])
        n96 = call "PPSU DC Off.vi"("Error in"=w197, "Device information"=w198) -> ("Error out"=w196:errorcluster)  [unwired: 8 in, 1 out]
      }
      frame "PPSU ACK Alarm " {
        n97 = Unbundle By Name(w199) -> ("Device information"=w200:string[])
        n98 = call "PPSU ACK alarm.vi"("Error in"=w202, "Device information arrayR"=w200) -> ("Error out"=w201:errorcluster)  [unwired: 8 in, 1 out]
      }
      frame "MS initialise" {
        n99 = Unbundle By Name(w203) -> ("Device information"=w204:string[])
        n100 = call "PPSU MS Init.vi"("Error in"=w206, "Device information arrayR"=w204) -> ("Fehler (Ausgang)"=w205:errorcluster)  [unwired: 8 in, 1 out]
      }
      frame "Exit" {
      }
      frame "Disable PPSU" {
        n101 = Unbundle By Name(w214) -> ("Device information"=w210:string[])
        n102 = Empty Array?(array=w210) -> (empty?=w213:bool)
        n103 = case shown="True" w213 {
          tunnel: [w219 w222] -> w212
          tunnel: w211 -> [w217 w222]
          tunnel: w210 -> [w215 _]
          frame False {
            n104 = call <vilib>:"Device_close.vi"("error in (no error)"=w217, "Device information in"=w215) -> ("Fehler (Ausgang)"=w216:errorcluster)  [unwired: 3 in]
            n105 = call "ALL HS.vi"("Loop"=ALL_Health."PPSU HS", "Option"=T5."Write '1'", "Status"=FALSE, "error in"=w216) -> ("error out"=w219:errorcluster)  [unwired: 9 in, 2 out]
          }
          frame True {
          }
        }
      }
    }
  }
  n106 = while {
    tunnel: w1 -> [w223]
    shift-right: [w224] -> _
    shift-left: Display_Loop_ctl."Motor" -> [w225]
    stop <- w226 stop-if-true
    # "Display loop"
    n107 = case shown="\"RTD\"" w225 {
      tunnel: [Display_Loop_ctl."RTD" Display_Loop_ctl."All Health" Display_Loop_ctl."PPSU" Display_Loop_ctl."Motor"] -> w224
      tunnel: w223 -> [_ _ _ _]
      frame "Motor", Default {
        w264 = enum16{"Read", "Write"}."Read" ("Enum")
        n108 = call "AI Voltage Current Data.vi"("Enum"=w264) -> ("AI Data"=w263:dbl[])  [unwired: 9 in, 1 out]
        n109 = Wait (ms)(milliseconds to wait=u32 100) -> ()  [unwired: 1 out]
        n110 = call "ETH_5 Data.vi"("Enum"=w264) -> ("Motor Feedback"=w275:T13)  [unwired: 9 in, 1 out]
        n111 = Index Array(array=w263) -> (element #1=→"Vab":dbl, element #2=→"Vbc":dbl, element #3=→"Vca":dbl, element #4=→"Ia":dbl, element #5=→"Ib":dbl, element #6=→"Ic":dbl, element #7=→"DAQ Idc":dbl, element #8=→"Ia_G":dbl, element #9=→"Ib_G":dbl, element #10=→"Ic_G":dbl, element #11=→"Idc_G":dbl, element #12=→"Vab_G":dbl, element #13=→"Vbc_G":dbl, element #14=→"Vca_G":dbl, element #15=→"Vdc_G":dbl, element #16=→"Vdc":dbl)  [unwired: 16 in]
        n112 = Unbundle By Name(w275) -> ("Run ACK"=→"RUN ACK":bool, "RDR"=→"RUN DUTY RATIO":dbl, "Sector"=→"SECTOR":dbl, "Halls Speed"=→"HALL SPEED":dbl, "Mode"=→"M-STATE FB":bool, "Voltage Speed"=→"VOLTAGE SPEED":dbl, "Direction"=→"DIRECTION":string, "IDC"=→"IDC":dbl, "Movable average"=→"Idc M-Avg":dbl, "VDC"=→"VDC":dbl)
        n113 = call "ETH_3 DATA.vi"("Enum"=enum16{"Read", "Write"}."Read") -> ("ETH 3"=w250:T13)  [unwired: 9 in, 1 out]
        n114 = call "DI Data.vi"("Enum"=enum16{"Write", "Read"}."Read") -> ("DI Data"=w261:bool[])  [unwired: 10 in]
        n115 = Unbundle By Name(w250) -> ("Run ACK"=→"RUN ACK":bool, "RDR"=→"RUN DUTY RATIO":dbl, "Sector"=→"SECTOR":dbl, "Halls Speed"=→"HALL SPEED":dbl, "Mode"=→"M-STATE FB":bool, "Voltage Speed"=→"VOLTAGE SPEED":dbl, "Direction"=→"DIRECTION":string, "IDC"=→"IDC":dbl, "Movable average"=→"Idc M-Avg":dbl, "VDC"=→"VDC":dbl)
        n116 = Index Array(array=w261) -> (element #1=→"Ha":bool, element #2=→"Hb":bool, element #3=→"Hc":bool, element #4=→"Ha_G":bool, element #5=→"Hb_G":bool, element #6=→"Hc_G":bool)  [unwired: 6 in]
      }
      frame "RTD" {
        n117 = call "ETH_4 Data.vi"("Enum"=enum16{"Read", "Write"}."Read") -> ("ETH_4"=w305:dbl[])  [unwired: 9 in, 1 out]
        n118 = call "ETH_2 Data.vi"("Enum"=enum16{"Read", "Write"}."Read") -> ("ETH_2"=w314:dbl[])  [unwired: 9 in, 1 out]
        n119 = Index Array(array=w305) -> (element #1=→"RTD  1":dbl, element #2=→"RTD  2":dbl, element #3=→"RTD  3":dbl, element #4=→"RTD  4":dbl, element #5=→"RTD  5":dbl, element #6=→"RTD  6":dbl)  [unwired: 6 in]
        n120 = Index Array(array=w314) -> (element #1=→"RTD  1":dbl, element #2=→"RTD  2":dbl, element #3=→"RTD 3":dbl, element #4=→"RTD  4":dbl, element #5=→"RTD  5":dbl, element #6=→"RTD 6":dbl)  [unwired: 7 in, 1 out]
        n121 = call "AI 20kHz data FGV.vi"("Enum"=enum16{"Read", "Write"}."Read") -> ("Propulsion Data"=w294:dbl[])  [unwired: 9 in, 1 out]
        n122 = Index Array(array=w294) -> (element #1=→"D_PT_1":dbl, element #2=→"D_PT_2":dbl, element #3=→"M_PT_1":dbl, element #4=→"IN_D_PT":dbl, element #5=→"D_RTD_1":dbl, element #6=→"D_RTD_2":dbl, element #7=→"M_RTD_1":dbl, element #8=→"OUT_D_RTD":dbl, element #9=→"IN_D_RTD":dbl, element #10=→"OUT_D_PT":dbl)  [unwired: 10 in]
        n123 = call "ETH_6.vi"("Enum"=enum16{"Read", "Write"}."Read") -> ("ETH_6"=w297:dbl[])  [unwired: 9 in, 1 out]
        n124 = Index Array(array=w297) -> (element #1=→"RTD  1":dbl, element #2=→"RTD  2":dbl, element #3=→"RTD  3":dbl, element #4=→"RTD  4":dbl, element #5=→"RTD  5":dbl, element #6=→"RTD  6":dbl)  [unwired: 6 in]
      }
      frame "All Health" {
        n125 = call "ALL HS.vi"("Option"=T5."Read 'All'") -> ("Status List Out"=w327:bool[])  [unwired: 12 in, 2 out]
        n126 = Index Array(array=w327) -> (element #1=→"AI HS":bool, element #2=→"AI 1kHZ HS":bool, element #3=→"AI 20kHZ HS":bool, element #4=→"DO HS":bool, element #5=→"LOG HS":bool, element #6=→"PPSU HS":bool, element #7=→"E1-MFB":bool, element #8=→"E1-RTD":bool, element #9=→"E2-MFB":bool, element #10=→"E2-RTD":bool, element #11=→"E5 - RTD":bool)  [unwired: 11 in]
      }
      frame "PPSU" {
        n127 = global read "6D_Global.vi" "T-Voltage"() -> (→"VOLTAGE":string)
        n128 = global read "6D_Global.vi" "T-Current"() -> (→"CURRENT":string)
        n129 = global read "6D_Global.vi" "T-Power"() -> (→"POWER":string)
        n130 = call "PPSU Detection.vi"("Write/Read"=enum16{"Write", "Read"}."Read") -> ("PPSU Dect"=w339:T14)  [unwired: 9 in, 1 out]
        n131 = Unbundle By Name(w339) -> ("Alarm"=→"PPSU Alarm":bool, "Power Fail"=→"Power Failure":bool, "OVD"=→"Over Voltage":bool, "OCD"=→"Over Current":bool, "OPD"=→"Over Power":bool, "MSP"=→"M-S Failure":bool)
      }
    }
    n132 = global read "6D_Global.vi" "Exit"() -> (w226:bool)
  }
  n133 = call "TCP_Receiver_Main.vi"("error in"=w1, "Queue Ref"=w2) -> ()  [unwired: 9 in, 1 out]
  n134 = call "D6 Datalog Main.vi"("error in"=w1, "Queue Ref"=w2) -> ()  [unwired: 10 in]
  n135 = call "DO Main.vi"("error In"=w1, "All Queue"=w2) -> ()  [unwired: 9 in, 1 out]
  n136 = call "AI DAQ.vi"("error in (no error)"=w1, "All Queue"=w2) -> ()  [unwired: 9 in, 1 out]
  n137 = call "AI Propulsion.vi"("error in (no error)"=w1, "All Queue"=w2) -> ()  [unwired: 10 in]
  n138 = while {
    tunnel: w1 -> [w347]
    tunnel: [w342] -> w14
    stop <- w341 stop-if-true
    # "Message Handler Loop"
    n139 = call "Main MH Queue.vi"("Option"=T7."DeQ", "error in (no error)"=w347) -> ("error out"=w346:errorcluster, "Message Out"=w345:cluster{"Message":string, "Data":variant})  [unwired: 8 in]
    n140 = Unbundle By Name(w345) -> ("Data"=w343:variant, "Message"=w344:string)
    n141 = case shown="\"Exit\"" w344 {
      tunnel: w346 -> [w349 w354 w373 w379 w383]
      tunnel: w343 -> [_ _ _ _ _]
      tunnel: [w349 w356 w372 w380 w383] -> w342
      tunnel: [_ _ _ _ TRUE] -> w341
      frame "", Default {
      }
      frame "Update E1A" {
        n142 = call "Connection Refnum.vi"("Option"=T5."Read '1'", "Loop"=Loop."ETH_1", "error in"=w354) -> ("ref  2"=w355:refnum<k5>, "error out"=w353:errorcluster)  [unwired: 10 in, 1 out]
        n143 = Cluster To Array(cluster="MOTOR") -> (array=w357:dbl[])
        n144 = for {
          tunnel: w357 -> [w365] mode=indexing
          tunnel: u8[] [18, 19, 20, 21, 22, 24] -> [w363] mode=indexing
          tunnel: w353 -> [w362]
          tunnel: [w361] -> w356
          tunnel: w355 -> [w359]
          n145 = call "Parameters to String.vi"("Input Data"=w365, "Packet Identifier"=w363) -> ("String"=w360:string)  [unwired: 9 in]
          n146 = TCP Write(connection ID=w359, data in=w360, error in (no error)=w362) -> (error out=w361:errorcluster)  [unwired: 1 in, 2 out]
          n147 = Wait (ms)(milliseconds to wait=u32 200) -> ()  [unwired: 1 out]
        }
      }
      frame "Motor On" {
        n148 = call "Parameters to String.vi"("Input Data"=1.0, "Packet Identifier"=u8 17) -> ("String"=w369:string)  [unwired: 9 in]
        n149 = call "Connection Refnum.vi"("Option"=T5."Read '1'", "Loop"=Loop."ETH_1") -> ("ref  2"=w367:refnum<k5>)  [unwired: 11 in, 2 out]
        n150 = TCP Write(connection ID=w367, data in=w369, error in (no error)=w373) -> (error out=w372:errorcluster)  [unwired: 1 in, 2 out]
      }
      frame "Motor Off" {
        n151 = call "Connection Refnum.vi"("Option"=T5."Read '1'", "Loop"=Loop."ETH_1") -> ("ref  2"=w378:refnum<k5>)  [unwired: 11 in, 2 out]
        n152 = call "Parameters to String.vi"("Input Data"=0.0, "Packet Identifier"=u8 17) -> ("String"=w376:string)  [unwired: 9 in]
        n153 = TCP Write(connection ID=w378, data in=w376, error in (no error)=w379) -> (error out=w380:errorcluster)  [unwired: 1 in, 2 out]
      }
      frame "Exit" {
      }
    }
  }
  n154 = while {
    tunnel: w1 -> [w386]
    tunnel: [w385] -> w13
    stop <- w384 stop-if-true
    # "Event Handler Loop"
    n155 = event shown="[1] \"DO CONFIG\": Value Change" {
      selector: _ -> [_ _ _ _ _ _ _ _ _ _ _ _ _ _ _ _ _ _ _ _ _ _ _ _ _ _ _ _ _]
      dyn-events: _ -> [_ _ _ _ _ _ _ _ _ _ _ _ _ _ _ _ _ _ _ _ _ _ _ _ _ _ _ _ _]
      timeout: _ -> [_ _ _ _ _ _ _ _ _ _ _ _ _ _ _ _ _ _ _ _ _ _ _ _ _ _ _ _ _]
      tunnel: w386 -> [w387 w389 w390 w398 _ _ w434 w444 w462 w477 w481 w490 w493 w503 w513 _ w531 w545 w547 w553 w559 w573 w577 w582 w587 w591 w605 w615 w627]
      tunnel: [w387 w389 w390 w393 _ _ w433 w443 w461 w470 w481 w489 w492 w502 w512 _ w530 w544 w546 w552 w559 w573 w577 w582 w587 w591 w605 w615 w621] -> w385
      tunnel: [_ _ _ _ _ _ _ _ _ _ _ _ _ _ _ _ _ _ _ _ FALSE _ FALSE _ _ _ _ _ TRUE] -> w384
      event Timeout {
        n156 = event-data() -> ()  [unwired: 1 in, 3 out]
      }
      event "DO CONFIG": Value Change {
        n157 = event-data() -> ("NewVal"=w388:cluster{"NAME":string, "CHANNEL NAME":tag}[])  [unwired: 1 in]
        n158 = global write "6D_Global.vi" "DO  Configuration"(w388) -> ()
      }
      event "Port Config File": Value Change {
        n159 = event-data() -> ()  [unwired: 1 in, 6 out]
        n160 = global write "6D_Global.vi" "Drive Config"("Port Config File") -> ()
      }
      event "Connect Drive": Value Change {
        n161 = event-data() -> ()  [unwired: 1 in, 6 out]
        n162 = call "Active Task FGV.vi"("Write/Read"=enum16{"Write", "Read"}."Write", "error in"=w398, "Activate Task"="Activate Task") -> ("error out"=w396:errorcluster)  [unwired: 7 in, 1 out]
        n163 = flat-sequence {
          tunnel: w396 -> [w401]
          tunnel: [w401] -> w395
          tunnel: [w400] -> w394
          tunnel: w395 -> [w404]
          tunnel: w394 -> [w405]
          tunnel: [w404] -> w393
          frame #0 {
            n164 = Two Button Dialog(message="Select Port Config", 1:"Select" ("F button name (\"Cancel\")"), 2:"Selected" ("T button name (\"OK\")")) -> (T button?=w400:bool)
          }
          frame #1 {
            n165 = case shown="True" w405 {
              frame False {
              }
              frame True {
                w406 = T10 [enum."Disabled and Grayed Out", enum."Enabled"] items=["Enabled", "Disabled", "Disabled and Grayed Out"] ("Disabled")
                n166 = control-ref of="Connect Drive"() -> (w408:refnum<vi>)
                n167 = control-ref of="Disconnect Drive"() -> (w409:refnum<vi>)
                n168 = call "Drive Status FGV.vi"("Disconnect Drive"=FALSE, "Connect Drive"=TRUE, "Enum"=enum16{"Read", "Write"}."Write") -> ()  [unwired: 6 in, 3 out]
                n169 = Build Array(w408, w409) -> (w407:refnum<vi>[])
                n170 = call "Enable ,Disable.vim"("Data"=w406, "Ref"=w407) -> ()  [unwired: 10 in]
              }
            }
          }
        }
      }
      event "Update RTD Offset": Value Change {
        n171 = event-data() -> ()  [unwired: 1 in, 6 out]
        n172 = call "ETH2_E1A_Offset.vi"("RTD1 Offset 1"="RTD 1 Offset", "RTD2 Offset"="RTD 2 Offset", "RTD3 Offset"="RTD 3 Offset", "RTD4 Offset"="RTD 4 Offset", "RTD5 Offset"="RTD 5 Offset", "RTD6 Offset"="RTD 6 Offset", "Write/Read"=enum16{"Write", "Read"}."Write") -> ()  [unwired: 7 in, 6 out]
        n173 = call "ETH2_E1A_Ref-V.vi"("Ref voltage"="V-Ref", "Write/Read"=enum16{"Write", "Read"}."Write") -> ()  [unwired: 9 in, 1 out]
      }
      event "Update RTD Offset_G": Value Change {
        w423 = enum16{"Write", "Read"}."Write" ("Write/Read")
        n174 = event-data() -> ()  [unwired: 1 in, 6 out]
        n175 = call "ETH4_E1L_Offset.vi"("RTD1 Offset 1"="RTD 1 Offset_G", "RTD2 Offset"="RTD 2 Offset_G", "RTD3 Offset"="RTD 3 Offset_G", "RTD4 Offset"="RTD 4 Offset_G", "RTD5 Offset"="RTD 5 Offset_G", "RTD6 Offset"="RTD 6 Offset_G", "Write/Read"=w423) -> ()  [unwired: 7 in, 6 out]
        n176 = call "ETH4_E1L_Ref-V.vi"("Ref voltage"="V-Ref_G", "Write/Read"=w423) -> ()  [unwired: 9 in, 1 out]
      }
      event "Update E1A": Value Change {
        n177 = event-data() -> ()  [unwired: 1 in, 1 out]
        n178 = Bundle By Name(cluster=cluster{"Message":string, "Data":variant} {"Message"="", "Data"=variant} ("Message"), "Message"="Update E1A") -> (w430:cluster{"Message":string, "Data":variant})
        n179 = call "Main MH Queue.vi"("Option"=T7."EnQ '1'", "error in (no error)"=w434, "Message"=w430) -> ("error out"=w433:errorcluster)  [unwired: 7 in, 1 out]
      }
      event "Motor On": Value Change {
        n180 = event-data() -> ("NewVal"=w436:bool)  [unwired: 1 in, 5 out]
        n181 = global read "6D_Global.vi" "DO Com"() -> (w442:bool[])
        n182 = Replace Array Subset(array=w442, new element=w436, index=1) -> (w441:bool[])
        n183 = global write "6D_Global.vi" "DO Com"(w441) -> ()
        n184 = Select(t="Motor On" ("Message"), s=w436, f="Motor Off" ("Message")) -> (s? t:f=w439:string)
        n185 = disable-structure shown="Enabled" {
          frame Disabled {
            w448 = T10 [enum."Disabled and Grayed Out", enum."Enabled"] items=["Enabled", "Disabled", "Disabled and Grayed Out"] ("Disabled")
            n186 = control-ref of="Motor On"() -> (w449:refnum<vi>)
            n187 = control-ref of="Motor Off"() -> (w450:refnum<vi>)
            n188 = Build Array(w449, w450) -> (w451:refnum<vi>[])
            n189 = call "Enable ,Disable.vim"("Data"=w448, "Ref"=w451) -> ()  [unwired: 10 in]
          }
          frame Enabled {
          }
        }
        n190 = Bundle By Name(cluster=cluster{"Message":string, "Data":variant} {"Message"="", "Data"=variant} ("Message"), "Message"=w439) -> (w447:cluster{"Message":string, "Data":variant})
        n191 = call "Main MH Queue.vi"("Option"=T7."EnQ '1'", "error in (no error)"=w444, "Message"=w447) -> ("error out"=w443:errorcluster)  [unwired: 7 in, 1 out]
      }
      event "Motor Off": Value Change {
        w457 = T10 [enum."Enabled", enum."Disabled and Grayed Out"] items=["Enabled", "Disabled", "Disabled and Grayed Out"] ("Disabled")
        n192 = event-data() -> ()  [unwired: 1 in, 6 out]
        n193 = property on="Motor Off" class="Bool (strict)"("Value"=FALSE ("Motor Off")) -> ()  [unwired: 2 in, 2 out]
        n194 = global read "6D_Global.vi" "DO Com"() -> (w455:bool[])
        n195 = Bundle By Name(cluster=cluster{"Message":string, "Data":variant} {"Message"="", "Data"=variant} ("Message"), "Message"="Motor Off") -> (w466:cluster{"Message":string, "Data":variant})
        n196 = Replace Array Subset(array=w455, new element=FALSE ("new element/subarray"), index=1) -> (w454:bool[])
        n197 = global write "6D_Global.vi" "DO Com"(w454) -> ()
        n198 = call "Main MH Queue.vi"("Option"=T7."EnQ '1'", "error in (no error)"=w462, "Message"=w466) -> ("error out"=w461:errorcluster)  [unwired: 7 in, 1 out]
        n199 = control-ref of="Motor On"() -> (w460:refnum<vi>)
        n200 = control-ref of="Motor Off"() -> (w459:refnum<vi>)
        n201 = Build Array(w460, w459) -> (w458:refnum<vi>[])
        n202 = call "Enable ,Disable.vim"("Data"=w457, "Ref"=w458) -> ()  [unwired: 10 in]
      }
      event "Disconnect Drive": Value Change {
        w473 = T10 [enum."Enabled", enum."Disabled and Grayed Out"] items=["Enabled", "Disabled", "Disabled and Grayed Out"] ("Disabled")
        n203 = event-data() -> ()  [unwired: 1 in, 6 out]
        n204 = call "Drive Status FGV.vi"("error in"=w477, "Disconnect Drive"=TRUE, "Connect Drive"=FALSE, "Enum"=enum16{"Read", "Write"}."Write") -> ("error out"=w472:errorcluster)  [unwired: 5 in, 2 out]
        n205 = call "Connection Refnum.vi"("Option"=T5."Read 'All'", "error in"=w472) -> ("ref  2"=w469:refnum<k5>, "error out"=w471:errorcluster)  [unwired: 11 in, 1 out]
        n206 = control-ref of="Connect Drive"() -> (w475:refnum<vi>)
        n207 = control-ref of="Disconnect Drive"() -> (w476:refnum<vi>)
        n208 = Build Array(w475, w476) -> (w474:refnum<vi>[])
        n209 = TCP Close Connection(connection ID=w469, abort (F)=TRUE, error in (no error)=w471) -> (error out=w470:errorcluster)  [unwired: 1 out]
        n210 = call "Enable ,Disable.vim"("Data"=w473, "Ref"=w474) -> ()  [unwired: 10 in]
      }
      event "PPSU IP": Value Change {
        n211 = event-data() -> ()  [unwired: 1 in, 6 out]
        n212 = global write "6D_Global.vi" "PPSU IP"("PPSU IP") -> ()
      }
      event "Enable PPSU": Value Change {
        n213 = event-data() -> ()  [unwired: 1 in, 6 out]
        n214 = Select(t="Enable PPSU" ("Message"), s="Enable PPSU", f="Disable PPSU" ("Message")) -> (s? t:f=w483:string)
        n215 = Bundle By Name(cluster=cluster{"Message":string, "Data":variant} {"Message"="", "Data"=variant} ("Message"), "Message"=w483) -> (w488:cluster{"Message":string, "Data":variant})
        n216 = call "PPSU Queue.vi"("Option"=T7."EnQ '1'", "error in"=w490, "Message"=w488) -> ("error out"=w489:errorcluster)  [unwired: 7 in, 1 out]
      }
      event "Update PPSU settings": Value Change {
        n217 = event-data() -> ()  [unwired: 1 in, 6 out]
        n218 = Bundle By Name(cluster=cluster{"Message":string, "Data":variant} {"Message"="", "Data"=variant} ("Message"), "Message"="Update PPSU settings") -> (w495:cluster{"Message":string, "Data":variant})
        n219 = call "PPSU Queue.vi"("Option"=T7."EnQ '1'", "error in"=w493, "Message"=w495) -> ("error out"=w492:errorcluster)  [unwired: 7 in, 1 out]
      }
      event "DC ON": Value Change {
        w498 = T10 [enum."Disabled and Grayed Out", enum."Enabled"] items=["Enabled", "Disabled", "Disabled and Grayed Out"] ("Disabled")
        n220 = event-data() -> ()  [unwired: 1 in, 6 out]
        n221 = Bundle By Name(cluster=cluster{"Message":string, "Data":variant} {"Message"="", "Data"=variant} ("Message"), "Message"="DC ON") -> (w507:cluster{"Message":string, "Data":variant})
        n222 = control-ref of="DC ON"() -> (w500:refnum<vi>)
        n223 = control-ref of="DC OFF"() -> (w501:refnum<vi>)
        n224 = call "PPSU Queue.vi"("Option"=T7."EnQ '1'", "error in"=w503, "Message"=w507) -> ("error out"=w502:errorcluster)  [unwired: 7 in, 1 out]
        n225 = Build Array(w500, w501) -> (w499:refnum<vi>[])
        n226 = call "Enable ,Disable.vim"("Data"=w498, "Ref"=w499) -> ()  [unwired: 10 in]
      }
      event "DC ON 2": Value Change {
        w510 = T10 [enum."Disabled and Grayed Out", enum."Enabled"] items=["Enabled", "Disabled", "Disabled and Grayed Out"] ("Disabled")
        n227 = event-data() -> ()  [unwired: 1 in, 6 out]
        n228 = Bundle By Name(cluster=cluster{"Message":string, "Data":variant} {"Message"="", "Data"=variant} ("Message"), "Message"="DC ON") -> (w514:cluster{"Message":string, "Data":variant})
        n229 = control-ref of="DC ON 2"() -> (w509:refnum<vi>)
        n230 = control-ref of="DC OFF 2"() -> (w508:refnum<vi>)
        n231 = call "PPSU 2 Queue.vi"("Option"=T7."EnQ '1'", "error in"=w513, "Message"=w514) -> ("error out"=w512:errorcluster)  [unwired: 7 in, 1 out]
        n232 = Build Array(w509, w508) -> (w511:refnum<vi>[])
        n233 = call "Enable ,Disable.vim"("Data"=w510, "Ref"=w511) -> ()  [unwired: 10 in]
      }
      event "Update RTD Offset_G 2": Value Change {
        w525 = enum16{"Write", "Read"}."Write" ("Write/Read")
        n234 = event-data() -> ()  [unwired: 1 in, 6 out]
        n235 = call "ETH6_E2A_Ref-V.vi"("Ref voltage"="V-Ref_B", "Write/Read"=w525) -> ()  [unwired: 9 in, 1 out]
        n236 = call "ETH6_E2A_Offset.vi"("RTD1 Offset 1"="RTD 1 Offset_B", "RTD2 Offset"="RTD 2 Offset_B", "RTD3 Offset"="RTD 3 Offset_B", "RTD4 Offset"="RTD 4 Offset_B", "RTD5 Offset"="RTD 5 Offset_B", "RTD6 Offset"="RTD 6 Offset_B", "Write/Read"=w525) -> ()  [unwired: 7 in, 6 out]
      }
      event "DC OFF": Value Change {
        w526 = T10 [enum."Enabled", enum."Disabled and Grayed Out"] items=["Enabled", "Disabled", "Disabled and Grayed Out"] ("Disabled")
        n237 = event-data() -> ()  [unwired: 1 in, 6 out]
        n238 = Bundle By Name(cluster=cluster{"Message":string, "Data":variant} {"Message"="", "Data"=variant} ("Message"), "Message"="DC OFF") -> (w535:cluster{"Message":string, "Data":variant})
        n239 = call "PPSU Queue.vi"("Option"=T7."EnQ '1'", "error in"=w531, "Message"=w535) -> ("error out"=w530:errorcluster)  [unwired: 7 in, 1 out]
        n240 = control-ref of="DC ON"() -> (w528:refnum<vi>)
        n241 = control-ref of="DC OFF"() -> (w529:refnum<vi>)
        n242 = Build Array(w528, w529) -> (w527:refnum<vi>[])
        n243 = call "Enable ,Disable.vim"("Data"=w526, "Ref"=w527) -> ()  [unwired: 10 in]
      }
      event "DC OFF 2": Value Change {
        w536 = T10 [enum."Disabled and Grayed Out", enum."Enabled"] items=["Enabled", "Disabled", "Disabled and Grayed Out"] ("Disabled")
        n244 = event-data() -> ()  [unwired: 1 in, 6 out]
        n245 = Bundle By Name(cluster=cluster{"Message":string, "Data":variant} {"Message"="", "Data"=variant} ("Message"), "Message"="DC OFF") -> (w540:cluster{"Message":string, "Data":variant})
        n246 = control-ref of="DC ON 2"() -> (w539:refnum<vi>)
        n247 = control-ref of="DC OFF 2"() -> (w538:refnum<vi>)
        n248 = Build Array(w538, w539) -> (w537:refnum<vi>[])
        n249 = call "PPSU 2 Queue.vi"("Option"=T7."EnQ '1'", "error in"=w545, "Message"=w540) -> ("error out"=w544:errorcluster)  [unwired: 7 in, 1 out]
        n250 = call "Enable ,Disable.vim"("Data"=w536, "Ref"=w537) -> ()  [unwired: 10 in]
      }
      event "PPSU ACK Alarm": Value Change {
        n251 = event-data() -> ()  [unwired: 1 in, 6 out]
        n252 = Bundle By Name(cluster=cluster{"Message":string, "Data":variant} {"Message"="", "Data"=variant} ("Message"), "Message"="PPSU ACK Alarm ") -> (w551:cluster{"Message":string, "Data":variant})
        n253 = call "PPSU Queue.vi"("Option"=T7."EnQ '1'", "error in"=w547, "Message"=w551) -> ("error out"=w546:errorcluster)  [unwired: 7 in, 1 out]
      }
      event "MS initialise": Value Change {
        n254 = event-data() -> ()  [unwired: 1 in, 6 out]
        n255 = Bundle By Name(cluster=cluster{"Message":string, "Data":variant} {"Message"="", "Data"=variant} ("Message"), "Message"="MS initialise") -> (w557:cluster{"Message":string, "Data":variant})
        n256 = call "PPSU Queue.vi"("Option"=T7."EnQ '1'", "error in"=w553, "Message"=w557) -> ("error out"=w552:errorcluster)  [unwired: 7 in, 1 out]
      }
      event "Start DAQ": Value Change {
        n257 = event-data() -> ()  [unwired: 1 in, 6 out]
        n258 = flat-sequence {
          frame #0 {
            n259 = Get Date/Time In Seconds() -> (seconds since 1Jan1904=w562:timestamp)
            n260 = Add(x=w562, y=15.0) -> (x+y=w561:timestamp)
            n261 = global write "6D_Global.vi" "Trigger"(w561) -> ()
          }
          frame #1 {
            w563 = T10 [enum."Disabled and Grayed Out", enum."Enabled"] items=["Enabled", "Disabled", "Disabled and Grayed Out"] ("Disabled")
            n262 = control-ref of="Start DAQ"() -> (w565:refnum<vi>)
            n263 = control-ref of="Stop DAQ"() -> (w564:refnum<vi>)
            n264 = global write "6D_Global.vi" "Start DAQ"(TRUE ("Start DAQ")) -> ()
            n265 = global write "6D_Global.vi" "Stop DAQ"(FALSE ("Stop DAQ")) -> ()
            n266 = Build Array(w565, w564) -> (w566:refnum<vi>[])
            n267 = call "Enable ,Disable.vim"("Data"=w563, "Ref"=w566) -> ()  [unwired: 10 in]
          }
        }
      }
      event "Stop DAQ": Value Change {
        w569 = T10 [enum."Enabled", enum."Disabled and Grayed Out"] items=["Enabled", "Disabled", "Disabled and Grayed Out"] ("Disabled")
        n268 = event-data() -> ()  [unwired: 1 in, 1 out]
        n269 = global write "6D_Global.vi" "Start DAQ"(FALSE ("Start DAQ")) -> ()
        n270 = global write "6D_Global.vi" "Stop DAQ"(TRUE ("Stop DAQ")) -> ()
        n271 = control-ref of="Start DAQ"() -> (w571:refnum<vi>)
        n272 = control-ref of="Stop DAQ"() -> (w570:refnum<vi>)
        n273 = Build Array(w571, w570) -> (w572:refnum<vi>[])
        n274 = call "Enable ,Disable.vim"("Data"=w569, "Ref"=w572) -> ()  [unwired: 10 in]
      }
      event "Continuous Log?": Value Change {
        n275 = event-data() -> ()  [unwired: 1 in, 6 out]
        n276 = global write "6D_Global.vi" "Contineous"(TRUE ("Contineous")) -> ()
      }
      event "Start Log": Value Change {
        w583 = T10 [enum."Disabled and Grayed Out", enum."Enabled"] items=["Enabled", "Disabled", "Disabled and Grayed Out"] ("Disabled")
        n277 = event-data() -> ()  [unwired: 1 in, 6 out]
        n278 = global write "6D_Global.vi" "Stop Log"(FALSE ("Stop Log")) -> ()
        n279 = global write "6D_Global.vi" "Start Log"(TRUE ("Start Log")) -> ()
        n280 = global write "6D_Global.vi" "Log Period"("Log Period") -> ()
        n281 = control-ref of="Start Log"() -> (w585:refnum<vi>)
        n282 = control-ref of="Stop Log"() -> (w584:refnum<vi>)
        n283 = Build Array(w585, w584) -> (w586:refnum<vi>[])
        n284 = call "Enable ,Disable.vim"("Data"=w583, "Ref"=w586) -> ()  [unwired: 10 in]
      }
      event "Datalog Prefix": Value Change {
        n285 = event-data() -> ()  [unwired: 1 in, 6 out]
        n286 = global write "6D_Global.vi" "Datalog Prefix"("Datalog Prefix") -> ()
      }
      event "Stop Log": Value Change {
        w592 = T10 [enum."Enabled", enum."Disabled and Grayed Out"] items=["Enabled", "Disabled", "Disabled and Grayed Out"] ("Disabled")
        n287 = event-data() -> ()  [unwired: 1 in, 6 out]
        n288 = global write "6D_Global.vi" "Start Log"(FALSE ("Start Log")) -> ()
        n289 = global write "6D_Global.vi" "Stop Log"(TRUE ("Stop Log")) -> ()
        n290 = control-ref of="Start Log"() -> (w594:refnum<vi>)
        n291 = control-ref of="Stop Log"() -> (w595:refnum<vi>)
        n292 = Build Array(w594, w595) -> (w593:refnum<vi>[])
        n293 = call "Enable ,Disable.vim"("Data"=w592, "Ref"=w593) -> ()  [unwired: 10 in]
      }
      event "GD ON": Value Change {
        w600 = T10 [enum."Disabled and Grayed Out", enum."Enabled"] items=["Enabled", "Disabled", "Disabled and Grayed Out"] ("Disabled")
        n294 = event-data() -> ()  [unwired: 1 in, 6 out]
        n295 = property on="GD ON" class="Bool (strict)"("Value"=FALSE ("GD ON")) -> ()  [unwired: 2 in, 2 out]
        n296 = control-ref of="GD ON"() -> (w598:refnum<vi>)
        n297 = control-ref of="GD OFF"() -> (w597:refnum<vi>)
        n298 = Build Array(w598, w597) -> (w599:refnum<vi>[])
        n299 = call "Enable ,Disable.vim"("Data"=w600, "Ref"=w599) -> ()  [unwired: 10 in]
        n300 = global read "6D_Global.vi" "DO Com"() -> (w604:bool[])
        n301 = Replace Array Subset(array=w604, new element=TRUE ("new element/subarray"), index=0) -> (w601:bool[])
        n302 = global write "6D_Global.vi" "DO Com"(w601) -> ()
      }
      event "GD OFF": Value Change {
        w607 = T10 [enum."Enabled", enum."Disabled and Grayed Out"] items=["Enabled", "Disabled", "Disabled and Grayed Out"] ("Disabled")
        n303 = event-data() -> ()  [unwired: 1 in, 6 out]
        n304 = control-ref of="GD ON"() -> (w609:refnum<vi>)
        n305 = control-ref of="GD OFF"() -> (w610:refnum<vi>)
        n306 = property on="GD OFF" class="Bool (strict)"("Value"=FALSE ("GD OFF")) -> ()  [unwired: 2 in, 2 out]
        n307 = Build Array(w609, w610) -> (w608:refnum<vi>[])
        n308 = call "Enable ,Disable.vim"("Data"=w607, "Ref"=w608) -> ()  [unwired: 10 in]
        n309 = global read "6D_Global.vi" "DO Com"() -> (w614:bool[])
        n310 = Replace Array Subset(array=w614, new element=FALSE ("new element/subarray"), index=0) -> (w611:bool[])
        n311 = global write "6D_Global.vi" "DO Com"(w611) -> ()
      }
      event "Exit": Value Change {
        n312 = event-data() -> ()  [unwired: 1 in, 6 out]
        n313 = Bundle By Name(cluster=cluster{"Message":string, "Data":variant} {"Message"="", "Data"=variant} ("Message"), "Message"="Exit") -> (w628:cluster{"Message":string, "Data":variant})
        n314 = global write "6D_Global.vi" "Exit"(TRUE ("Exit")) -> ()
        n315 = call "Main MH Queue.vi"("Option"=T7."EnQ Opp", "error in (no error)"=w627, "Message"=w628) -> ("error out"=w622:errorcluster)  [unwired: 7 in, 1 out]
        n316 = Bundle By Name(cluster=cluster{"Message":string, "Data":variant} {"Message"="", "Data"=variant} ("Message"), "Message"="Exit") -> (w626:cluster{"Message":string, "Data":variant})
        n317 = call "PPSU Queue.vi"("Option"=T7."EnQ Opp", "error in"=w622, "Message"=w626) -> ("error out"=w620:errorcluster)  [unwired: 7 in, 1 out]
        n318 = Bundle By Name(cluster=cluster{"Message":string, "Data":variant} {"Message"="", "Data"=variant} ("Message"), "Message"="Exit") -> (w616:cluster{"Message":string, "Data":variant})
        n319 = call "PPSU 2 Queue.vi"("Option"=T7."EnQ Opp", "error in"=w620, "Message"=w616) -> ("error out"=w621:errorcluster)  [unwired: 7 in, 1 out]
      }
    }
  }
  n320 = call "PPSU Feedback.vi"("Error in"=w1, "All Queue"=w2) -> ()  [unwired: 10 in]
  n321 = disable-structure shown="Disabled" {
    frame Disabled {
      n322 = stacked-sequence {
        tunnel: _ -> [w634 _ _]
        tunnel: [w634 _ _] -> _
        frame #0 {
          n323 = global read "6D_Global.vi" "DO Com"() -> (w638:bool[])
          n324 = Replace Array Subset(array=w638, new element=TRUE ("new element/subarray"), index=0) -> (w635:bool[])
          n325 = global write "6D_Global.vi" "DO Com"(w635) -> ()
        }
        frame #1 {
          n326 = Wait (ms)(milliseconds to wait=u32 500) -> ()  [unwired: 1 out]
        }
        frame #2 {
          n327 = global read "6D_Global.vi" "DO Com"() -> (w642:bool[])
          n328 = Replace Array Subset(array=w642, new element=FALSE ("new element/subarray"), index=0) -> (w643:bool[])
          n329 = global write "6D_Global.vi" "DO Com"(w643) -> ()
        }
      }
    }
    frame Enabled {
    }
  }
  n330 = Merge Errors(w13, w14, w17) -> (w19:errorcluster)
  n331 = call <vilib>:"Clear Errors.vi"("error in (no error)"=w19) -> ()  [unwired: 5 in, 2 out]
